vi "Trigger Measurement.vi"(0 "Ratio Two Channels \n(Enable V1/V2 Measure)":bool, 8 "VISA resource name":refnum<visa-resource-name>="GPIB0::5::INSTR", 11 "milliseconds to wait":u32=2500) -> (1 "Standard Deviation":dbl, 2 "Mean":dbl=1.0, 3 "Buffer":ext[](array[numeric]) format="%#_10g")   [LabVIEW 2011]
uses:
  Documents/Keithley 2182/Keithley 2182.lvlib
panel:
  in  "Selected Calculation Settings":enum32{"Linear Settings", "Percent Settings"}(tab)
  out "Buffer Metadata":T1(array[cluster])
  out "Maximum":dbl
  out "Minimum":dbl
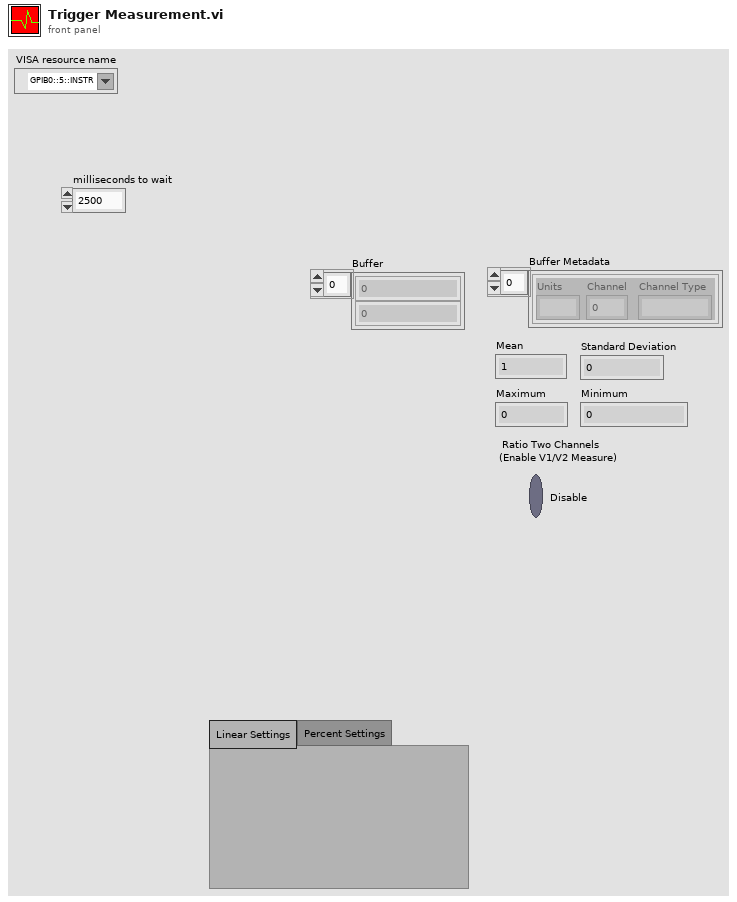
[diagram p1: front panel]
types:
  T1 = cluster{"Units":string, "Channel":i32, "Channel Type":string}[]
  T2 = enum32{"Voltage Settings", "Temperature Settings"}
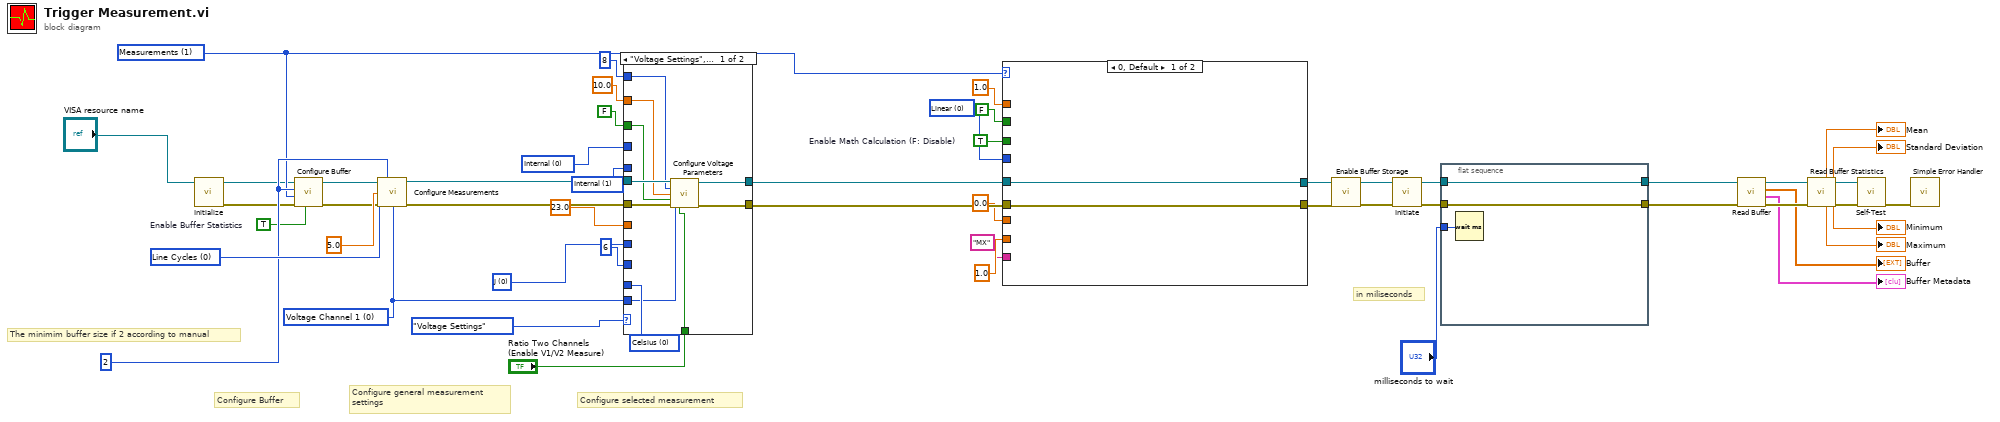
[diagram p0: block diagram]
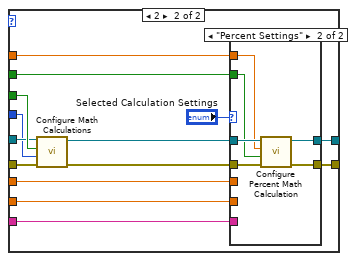
[diagram p2: hidden frame]
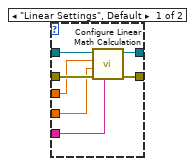
[diagram p3: hidden frame]
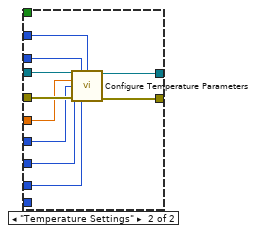
[diagram p4: hidden frame]
diagram:
  w27 = 0 items=["Linear", "Percent"] ("Math Calculation (0: Linear)")
  w35 = 0 items=["Celsius", "Fahrenheit", "Kelvin"] ("Unit (0: Celsius)")
  w33 = 0 items=["J", "K", "T", "E", "R", "S", "B", "N"] ("Thermocouple Type (0: J)")
  w30 = 0 items=["Internal", "Simulated"] ("Reference Junction Type (0: Internal)")
  w31 = 1 items=["Thermocouple", "Internal"] ("Sensor (1: Internal)")
  w16 = 0 items=["Voltage Channel 1", "Voltage Channel 2", "Temperature Channel 1", "Temperature Channel 2"] ("Measurement (0: Voltage Channel 1)")
  w44 = 0 items=["Line Cycles", "Seconds"] ("Integration Rate Units (0: Line Cycles)")
  w41 = 2 ("Buffer Size (10)")
  w29 = 1 items=["None", "Measurements", "Math Calculation"] ("Buffer Source (0: None)")
  w6 = TRUE  # Enable Buffer Statistics
  w28 = TRUE  # Enable Math Calculation (F: Disable)
  # "in miliseconds"
  # "The minimim buffer size if 2 according to manual"
  # "Configure general measurement\nsettings"
  # "Configure Buffer"
  # "Configure selected measurement"
  n1 = call "Initialize.vi"("VISA resource name"="VISA resource name") -> ("error out"=w19:errorcluster, "VISA resource name out"=w18:refnum<visa-resource-name>)  [unwired: 9 in]
  n2 = call "Configure Buffer.vi"("Enable Buffer Statistics (0: Disable)"=w6, "error in (no error)"=w19, "Buffer Source (0: None)"=w29, "Buffer Size (2)"=w41, "VISA resource name"=w18) -> ("error out"=w43:errorcluster, "VISA resource name out"=w42:refnum<visa-resource-name>)  [unwired: 5 in]
  n3 = call "Configure Measurements.vi"("VISA resource name"=w42, "Measurement (0: Voltage Channel 1)"=w16, "Integration Rate (5)"=5.0, "Integration Rate Units (0: Line Cycles)"=w44, "error in (no error)"=w43, "Sample Count (1)"=w41) -> ("VISA resource name out"=w36:refnum<visa-resource-name>, "error out"=w37:errorcluster)  [unwired: 8 in]
  n4 = case shown="\"Voltage Settings\", Default" T2."Voltage Settings" ("Selected Measurement Settings") {
    tunnel: 8 ("Voltage Resolution (8)") -> [w56 _]
    tunnel: 10.0 ("Range Value (10)") -> [w57 _]
    tunnel: FALSE ("Autorange (T: Enable)") -> [w58 _]
    tunnel: w37 -> [w62 w72]
    tunnel: w36 -> [w61 w71]
    tunnel: [w60 w70] -> w25
    tunnel: [w59 w69] -> w26
    tunnel: w35 -> [_ w68]
    tunnel: 6 ("Temperature Resolution (6)") -> [_ w67]
    tunnel: w33 -> [_ w66]
    tunnel: 23.0 ("Simulated Reference Temp (23 C)") -> [_ w65]
    tunnel: w31 -> [_ w64]
    tunnel: w30 -> [_ w63]
    tunnel: w16 -> [w55 _]
    tunnel: "Ratio Two Channels \n(Enable V1/V2 Measure)" -> [w54 _]
    frame "Voltage Settings", Default {
      n5 = call "Configure Voltage Parameters.vi"("VISA resource name"=w61, "Measurement (1: Voltage Channel 1)"=w55, "Voltage Resolution (8)"=w56, "Range Value (12)"=w57, "Autorange (T: Enable)"=w58, "error in (no error)"=w62, "Enable Ratio (F: Disable)"=w54) -> ("VISA resource name out"=w60:refnum<visa-resource-name>, "error out"=w59:errorcluster)  [unwired: 7 in]
    }
    frame "Temperature Settings" {
      n6 = call "Configure Temperature Parameters.vi"("VISA resource name"=w71, "Sensor (0: Thermocouple)"=w64, "Reference Junction Type (0: Internal)"=w63, "Simulated Reference Temp (23 C)"=w65, "Thermocouple Type (0: J)"=w66, "Temperature Resolution (6)"=w67, "error in (no error)"=w72, "Unit (0: Celsius)"=w68) -> ("VISA resource name out"=w70:refnum<visa-resource-name>, "error out"=w69:errorcluster)  [unwired: 6 in]
    }
  }
  n7 = case shown="0, Default" w29 {
    tunnel: w28 -> [_ w88]
    tunnel: w27 -> [_ w85]
    tunnel: w26 -> [w74 w87]
    tunnel: w25 -> [w73 w86]
    tunnel: FALSE ("Use Input Signal as Target Value (F: Disable)") -> [_ w84]
    tunnel: 1.0 ("Target Value (1)") -> [_ w83]
    tunnel: 0.0 ("Offset Value (0)") -> [_ w80]
    tunnel: 1.0 ("Scale Factor (1)") -> [_ w79]
    tunnel: "MX" ("Units (MX)") -> [_ w78]
    tunnel: [w74 w77] -> w15
    tunnel: [w73 w76] -> w12
    frame 0, Default {
    }
    frame 2 {
      n8 = call "Configure Math Calculations.vi"("error in (no error)"=w87, "Math Calculation (0: Linear)"=w85, "Enable Math Calculation (F: Disable)"=w88, "VISA resource name"=w86) -> ("error out"=w82:errorcluster, "VISA resource name out"=w81:refnum<visa-resource-name>)  [unwired: 6 in]
      n9 = case shown="\"Percent Settings\"" "Selected Calculation Settings" {
        tunnel: w84 -> [_ w97]
        tunnel: w83 -> [_ w96]
        tunnel: w82 -> [w95 w98]
        tunnel: w81 -> [w94 w99]
        tunnel: w80 -> [w93 _]
        tunnel: w79 -> [w92 _]
        tunnel: w78 -> [w91 _]
        tunnel: [w90 w101] -> w77
        tunnel: [w89 w100] -> w76
        frame "Linear Settings", Default {
          n10 = call "Configure Linear Math Calculation.vi"("Units (MX)"=w91, "error in (no error)"=w95, "Offset Value (0)"=w92, "Scale Factor (1)"=w93, "VISA resource name"=w94) -> ("error out"=w90:errorcluster, "VISA resource name out"=w89:refnum<visa-resource-name>)  [unwired: 5 in]
        }
        frame "Percent Settings" {
          n11 = call "Configure Percent Math Calculation.vi"("error in (no error)"=w98, "Use Input Signal as Target Value (F: Disable)"=w97, "Target Value (1)"=w96, "VISA resource name"=w99) -> ("error out"=w101:errorcluster, "VISA resource name out"=w100:refnum<visa-resource-name>)  [unwired: 6 in]
        }
      }
    }
  }
  n12 = call "Enable Buffer Storage.vi"("error in (no error)"=w15, "VISA resource name"=w12) -> ("error out"=w14:errorcluster, "VISA resource name out"=w13:refnum<visa-resource-name>)  [unwired: 8 in]
  n13 = call "Initiate.vi"("error in (no error)"=w14, "VISA resource name"=w13) -> ("error out"=w9:errorcluster, "VISA resource name out"=w7:refnum<visa-resource-name>)  [unwired: 8 in]
  n14 = flat-sequence {
    tunnel: "milliseconds to wait" -> [w104]
    tunnel: [w103] -> w10
    tunnel: w9 -> [w103]
    tunnel: [w102] -> w8
    tunnel: w7 -> [w102]
    frame #0 {
      n15 = Wait (ms)(milliseconds to wait=w104) -> ()  [unwired: 1 out]
    }
  }
  n16 = call "Read Buffer.vi"("error in (no error)"=w10, "VISA resource name"=w8) -> ("error out"=w52:errorcluster, "Buffer Metadata"=→"Buffer Metadata":T1, "Buffer"=→"Buffer":ext[], "VISA resource name out"=w51:refnum<visa-resource-name>)  [unwired: 6 in]
  n17 = call "Read Buffer Statistics.vi"("error in (no error)"=w52, "VISA resource name"=w51) -> ("error out"=w5:errorcluster, "Minimum"=→"Minimum":dbl, "Standard Deviation"=→"Standard Deviation":dbl, "VISA resource name out"=w4:refnum<visa-resource-name>, "Maximum"=→"Maximum":dbl, "Mean"=→"Mean":dbl)  [unwired: 4 in]
  n18 = call "Self-Test.vi"("error in (no error)"=w5, "VISA resource name"=w4) -> ("error out"=w3:errorcluster)  [unwired: 6 in, 3 out]
  n19 = call <vilib>:"Simple Error Handler.vi"("error in (no error)"=w3) -> ()  [unwired: 4 in, 5 out]
